vi "Timer.vi"() -> ()   [LabVIEW 2019]
uses:
  <vilib>/Platform/TimedLoop/XDataNode/timing_clust.ctl
  <vilib>/Platform/TimedLoop/XDataNode/nitl_modes.ctl
  <vilib>/Platform/TimedLoop/XDataNode/wakeup.ctl
  <vilib>/platform/TimedLoop/XDataNode/XDataNode.xnode
  <vilib>/Platform/TimedLoop/XDataNode/XDNodeRunTimeDep.lvlib
panel:
  out "Timer":dbl
  out "x >= y?":bool
  out "Second Time":dbl caption="Second"
  out "StartTime":dbl caption="Start"
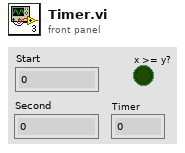
[diagram p1: front panel]
types:
  T1 = typedef "XDNodeRunTimeDep.lvlib/timing_clust.ctl" = cluster{"Expected End [f-1]":u64, "Actual End [f-1]":u64, "Finished Late? [f-1]":bool, "Expected End [i-1]":u64, "Actual End [i-1]":u64, "Finished Late? [i-1]":bool, "Expected Start [i]":u64, "Actual Start [i]":u64, "Expected Start [f]":u64, "Actual Start [f]":u64, "Source Name":string, "Structure Name":string, "Period":i64, "Deadline":i64, "Offset":i64, "Start":i64, "Priority":i32, "Timeout":i32, "Mode":T2, "Wakeup Reason":T3, "Error":errorcluster, "Source Type":string, "Secondary Source Type":string, "Global End Time":u64, "Global Start Time":u64, "Frame Duration":u64, "Iteration Duration":u64, "Assigned CPU":i32, "I/O Scan Engine Mode":u32}
  T2 = typedef "XDNodeRunTimeDep.lvlib/nitl_modes.ctl" = enum32{"No Change", "Process missed periods, maintain original phase", "Discard missed periods, maintain original phase", "Process missed periods, ignore original phase", "Discard missed periods, ignore original phase"}
  T3 = typedef "XDNodeRunTimeDep.lvlib/wakeup.ctl" = enum32{"Normal", "Aborted", "Asynchronous wakeup", "Timing source error", "Timed loop error", "Timeout"}
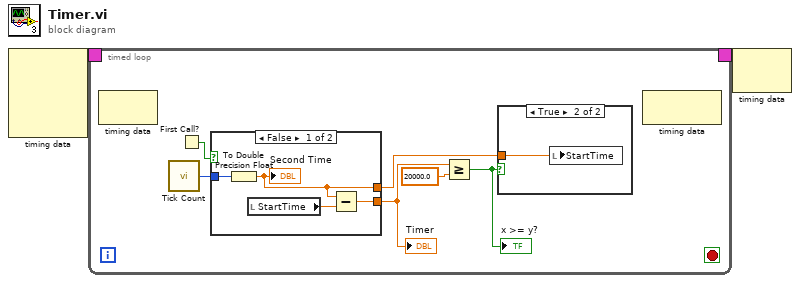
[diagram p0: block diagram]
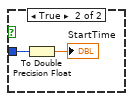
[diagram p3: hidden frame]
diagram:
  n1 = node-c288() -> (w2:T1)  [unwired: 4 in]
  n2 = timed-loop {
    timing: w2 -> [_]
    timing-out: [_] -> w1
    stop <- _ stop-if-true
    n3 = node-c288() -> ()  [unwired: 1 in, 1 out]
    n4 = call "Tick Count"() -> ("Tick Count(mSec)"=w5:u32)
    n5 = First Call?() -> (First Call?: T/F=w8:bool)
    n6 = case shown="False" w8 {
      tunnel: [w12 _] -> w7
      tunnel: w5 -> [w11 w15]
      tunnel: [w10 _] -> w4
      frame False {
        n7 = To Double Precision Float(number=w11) -> (double precision float=w10:dbl)
        "Second Time" <- w10
        n8 = local read "StartTime"() -> (w13:dbl)
        n9 = Subtract(x=w10, y=w13) -> (x-y=w12:dbl)
      }
      frame True {
        n10 = To Double Precision Float(number=w15) -> (double precision float=→"StartTime":dbl)
      }
    }
    "Timer" <- w7
    n11 = Greater Or Equal?(x=w7, y=20000.0) -> (x >= y?=w3:bool)
    "x >= y?" <- w3
    n12 = case shown="True" w3 {
      tunnel: w4 -> [_ w9]
      frame False {
      }
      frame True {
        n13 = local write "StartTime"(w9) -> ()
      }
    }
    n14 = node-c288() -> ()  [unwired: 1 in, 1 out]
  }
  n15 = node-c288(w1) -> ()  [unwired: 1 out]
